vi "boolean to U8.vi"(11 "Boolean array in":bool[][](array[boolean])) -> (3 "Array out":i32[][](array[numeric]))   [LabVIEW 2016]
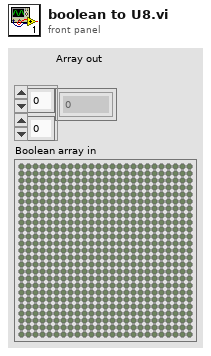
[diagram p1: front panel]
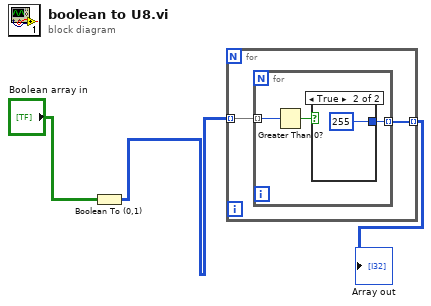
[diagram p0: block diagram]
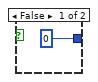
[diagram p2: hidden frame]
diagram:
  n1 = Boolean To (0,1)(Boolean="Boolean array in") -> (0, 1=w1:i16[][])
  n2 = for {
    tunnel: w1 -> [w5] mode=indexing
    tunnel: [w4] -> w3 mode=indexing
    n3 = for {
      tunnel: w5 -> [w7] mode=indexing
      tunnel: [w6] -> w4 mode=indexing
      n4 = Greater Than 0?(x=w7) -> (x > 0?=w8:bool)
      n5 = case shown="True" w8 {
        tunnel: [0 255] -> w6
        frame False {
        }
        frame True {
        }
      }
    }
  }
  "Array out" <- w3
